vi "AfterPage2_GenCDP.vi"(10 "MetaDataObj":refnum<class "MetaDataObj.lvclass">, 11 "User Project":refnum<vi>) -> ()   [LabVIEW 2026, in "NIVS_CDEW_MetaDataObj.lvclass"]
uses:
  NIVS_CDEW_MetaDataObj.lvclass
  <resource>/dialog/NewProjectWizard/MetaDataObj/MetaDataObj.lvclass
  NIVS_CDEW_MetaDataObj.lvclass/NIVS_CDEW_MetaDataObj.ctl
  <resource>/dialog/NewProjectWizard/MetaDataObj/MetaDataObj.lvclass/MetaDataObj.ctl
  <resource>/dialog/NewProjectWizard/MetaDataObj/Accessors/Read Project Root.vi
  <resource>/dialog/NewProjectWizard/MetaDataObj/Accessors/Read Project Name.vi
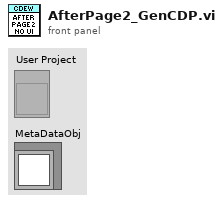
[diagram p1: front panel]
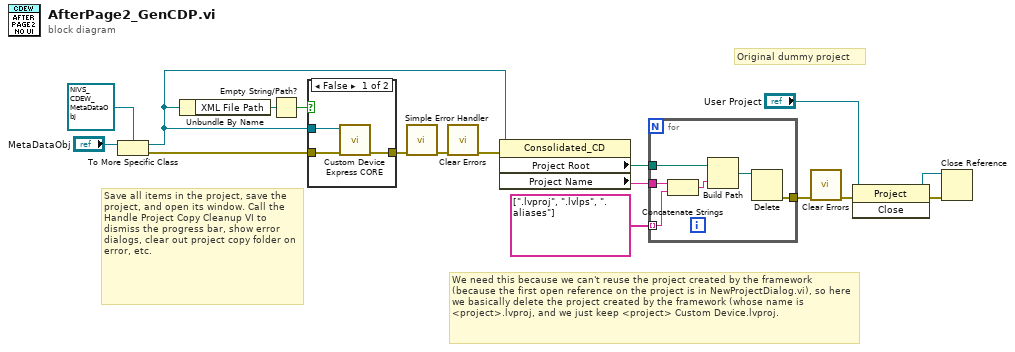
[diagram p0: block diagram]
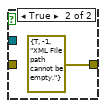
[diagram p2: hidden frame]
diagram:
  # "Original dummy project"
  # "We need this because we can't reuse the project created by the framework (because the first open reference on the project is in NewProjectDialog.vi), so here we basically delete the project created by the framework (whose name is <project>.lvproj, and we just keep <project> Custom Device.lvproj."
  # "Save all items in the project, save the project, and open its window. Call the Handle Project Copy Cleanup VI to dismiss the progress bar, show error dialogs, clear out project copy folder on error, etc."
  n1 = To More Specific Class(target class=refnum<class "NIVS_CDEW_MetaDataObj.lvclass"> refnum ("NIVS_CDW_MetaDataObj.lvclass"), reference="MetaDataObj") -> (specific class reference=w3:refnum<class "NIVS_CDEW_MetaDataObj.lvclass">, error out=w16:errorcluster)  [unwired: 1 in]
  n2 = Unbundle By Name(w3) -> ("XML File Path"=w6:path)
  n3 = Empty String/Path?(string/path=w6) -> (empty?=w5:bool)
  n4 = case shown="False" w5 {
    tunnel: w16 -> [w20 _]
    tunnel: [w19 errorcluster {"status"=TRUE, "code"=-1, "source"="XML File path cannot be empty."} ("error in (no error)")] -> w2
    tunnel: w3 -> [w18 _]
    frame False {
      n5 = call "Custom Device Express CORE.vi"("error in"=w20, "CDEW_MetaDataObj"=w18) -> ("error out"=w19:errorcluster)  [unwired: 8 in, 1 out]
    }
    frame True {
    }
  }
  n6 = call <vilib>:"Simple Error Handler.vi"("error in (no error)"=w2) -> ("error out"=w1:errorcluster)  [unwired: 4 in, 4 out]
  n7 = call <vilib>:"Clear Errors.vi"("error in (no error)"=w1) -> ("error out"=w7:errorcluster)  [unwired: 5 in, 1 out]
  n8 = property class="Consolidated_CD"(reference=w3, error in=w7) -> ("Project Root"=w15:path, "Project Name"=w14:string)  [unwired: 2 out]
  n9 = for {
    tunnel: w15 -> [w27]
    tunnel: w14 -> [w26]
    tunnel: string[] [".lvproj", ".lvlps", ".aliases"] -> [w25] mode=indexing
    tunnel: [w22] -> w12
    n10 = Concatenate Strings(w26, w25) -> (w24:string)
    n11 = Build Path(base path=w27, name or relative path=w24) -> (appended path=w23:path)
    n12 = Delete(path (use dialog)=w23) -> (error out=w22:errorcluster)  [unwired: 4 in, 2 out]
  }
  n13 = call <vilib>:"Clear Errors.vi"("error in (no error)"=w12) -> ("error out"=w11:errorcluster)  [unwired: 5 in, 1 out]
  n14 = invoke class="Project" method="Close"(reference="User Project", error in=w11) -> (reference out=w8:refnum<vi>, error out=w9:errorcluster)  [unwired: 1 in, 1 out]
  n15 = Close Reference(reference=w8, error in (no error)=w9) -> ()  [unwired: 1 out]
